vi "generate empty sample array.vi"(11 "Numeric":u32) -> (3 "output cluster":T1)   [LabVIEW 2014]
uses:
  Controls/Audio In.ctl
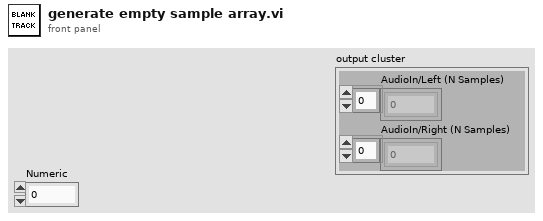
[diagram p1: front panel]
types:
  T1 = typedef "Audio In.ctl" = cluster{"AudioIn/Left (N Samples)":dbl[], "AudioIn/Right (N Samples)":dbl[]}
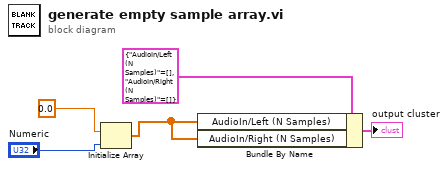
[diagram p0: block diagram]
diagram:
  n1 = Initialize Array(0.0, "Numeric") -> (w3:dbl[])
  n2 = Bundle By Name(cluster=T1 {"AudioIn/Left (N Samples)"=[], "AudioIn/Right (N Samples)"=[]} ("Track 3"), "AudioIn/Left (N Samples)"=w3, "AudioIn/Right (N Samples)"=w3) -> (→"output cluster":T1)
